vi "Basic TESTER.vi"() -> ()   [LabVIEW 2020]
uses:
  <vilib>/Rock Robotics/WPI/ThirdParty/Phoenix-LabVIEW/Pigeon IMU/CTRE_PigeonIMU_StatusFrameRate.ctl
  <vilib>/Rock Robotics/WPI/ThirdParty/Phoenix-LabVIEW/Pigeon IMU/CTRE_PigeonIMU_GetYPR.vi
  SwerveDrive/SwerveDrive_ACT.lvlib
  <vilib>/Rock Robotics/WPI/ThirdParty/Phoenix-LabVIEW/Pigeon2/controls/CTRE_Phoenix_Pigeon2_Configurables.ctl
  <vilib>/Rock Robotics/WPI/ThirdParty/Phoenix-LabVIEW/Pigeon IMU/CTRE_PigeonIMU_TareType.ctl
  Shared Code/TypeDefs/Dial_Compase heading unit circle CCW positive.ctl
panel:
  out "Yaw Angle":T1 scale format="%.3f"
  in  "Value":dbl format="%#_13g"
  in  "TareType (SetValue)":T2=2 items=["SetValue"=0, "AddOffset"=1, "MatchCompass"=2, "SetOffset"=255]
  in  "Set Yaw":bool
  out "error out":errorcluster
  out "periodMs":u32
  out "Has Reset Occurred?":bool
  out "Numeric":i32
  out "Yaw Pitch Roll":cluster{"Yaw":dbl, "Pitch":dbl, "Roll":dbl}
  out "firmware version":i32
  in  "Pigeon2 Configurables":T3
  in  "Finish":bool
  # "Pitch Angle needed to reach the current orientation in degrees"
  # "Yaw Angle needed to reach the current orientation in degrees"
  # "Configures the mounting pose of the Pigeon2\nThis is the yaw-pitch-roll teh Pigeon2 underwent to get to its current orientation,\n referenced from the robot's point of view\nThis is only necessary if the Pigeon2 is mounted at an exotic angle near the gimbal lock point or not forward.\nIf the pigeon is relatively flat and pointed forward, this is not needed"
  # "Roll Angle needed to reach the current orientation in degrees"
  # "Disables the temperature compensation\nfrom the Pigeon2. It is recommended that\nthis remains false"
  # "Disables the no-motion calibration from the\nPigeon2. It is recommended that this \nremains false"
  # "Enables the compass for Pigeon2\nThis is not recommended for any indoor robotics"
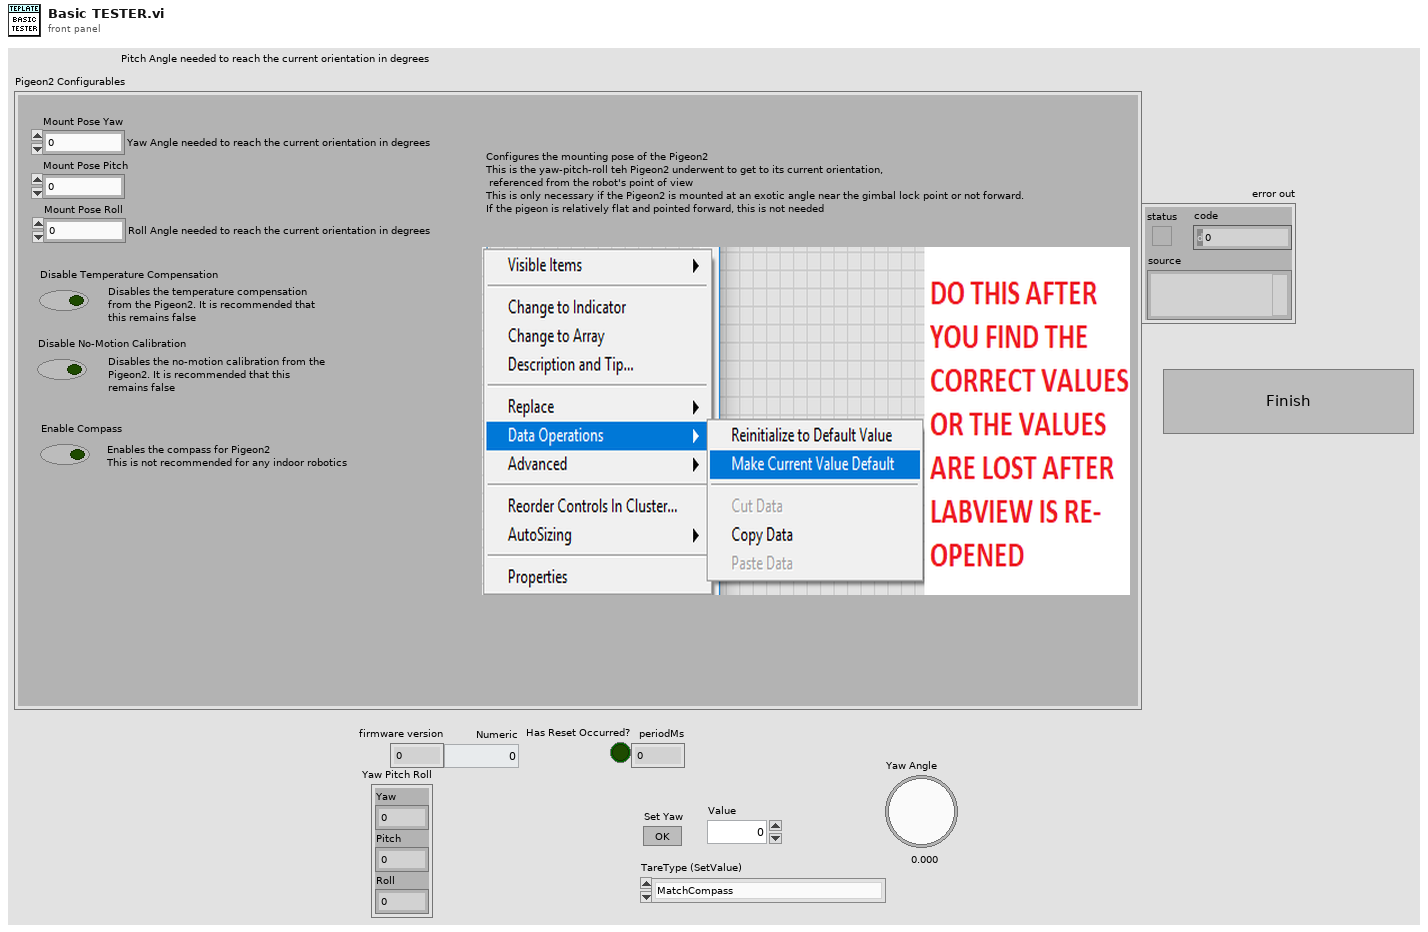
[diagram p1: front panel]
types:
  T1 = typedef "Dial_Compase heading unit circle CCW positive.ctl" = dbl
  T2 = typedef "CTRE_PigeonIMU_TareType.ctl" = u8
  T3 = typedef "CTRE_Phoenix_Pigeon2_Configurables.ctl" = cluster{"Mount Pose Yaw":dbl, "Mount Pose Pitch":dbl, "Mount Pose Roll":dbl, "Disable Temperature Compensation":bool, "Disable No-Motion Calibration":bool, "Enable Compass":bool}
  T4 = typedef "CTRE_PigeonIMU_DeviceRef.ctl" = cluster{"DeviceStatus":errorcluster, "Device Number":u8, "Type":T5, "Device ID":u32, "Handle":u64, "UsageFrame":u32, "Library Path":path}
  T5 = typedef "CTRE_PigeonIMU_ConnectionType.ctl" = u32
  T6 = typedef "CTRE_PigeonIMU_StatusFrameRate.ctl" = u32
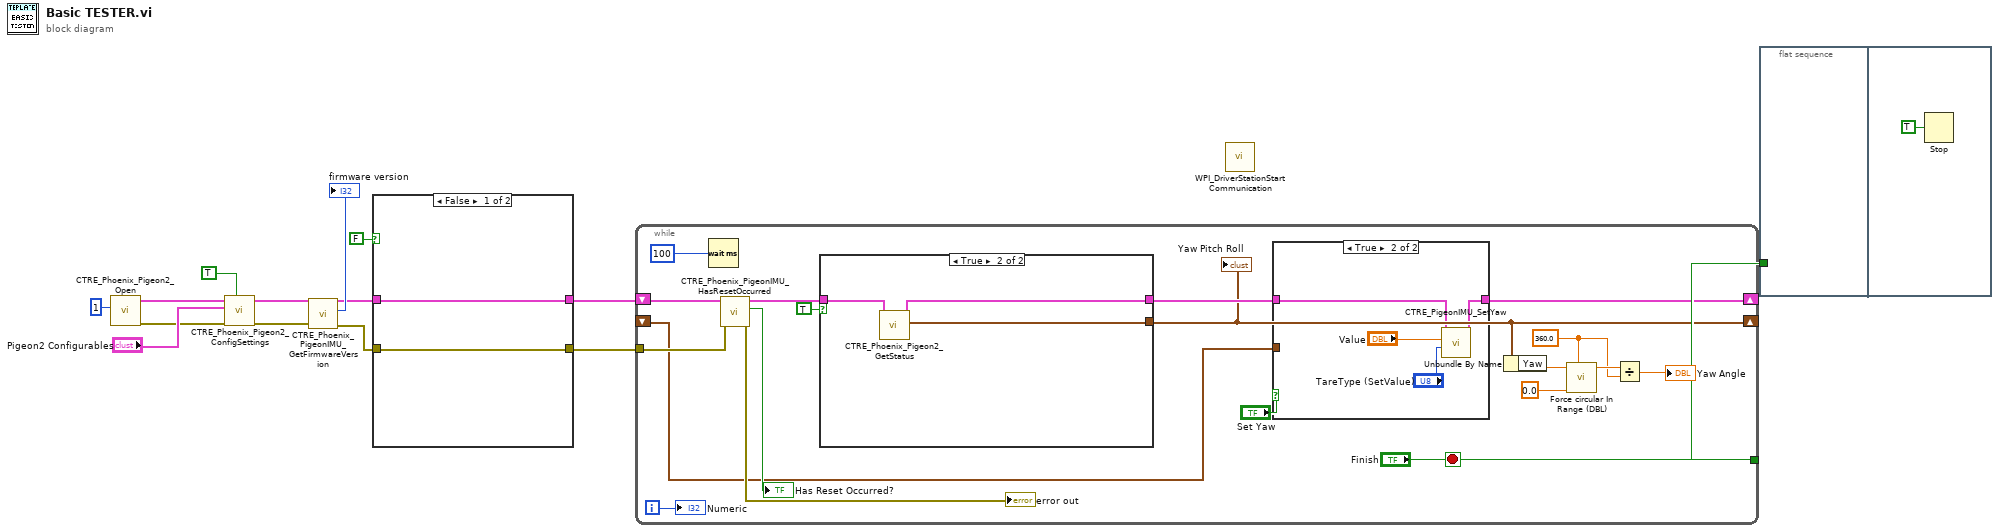
[diagram p0: block diagram]
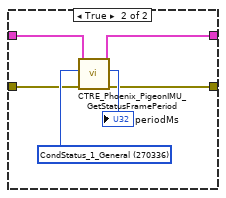
[diagram p2: hidden frame]
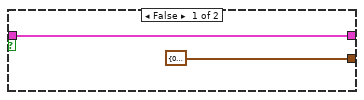
[diagram p4: hidden frame]
diagram:
  n1 = call <vilib>:"CTRE_Phoenix_Pigeon2_Open.vi"("Device Number"=u8 1) -> ("error out"=w5:errorcluster, "PigeonIMUDevRef"=w12:T4)  [unwired: 9 in]
  n2 = call <vilib>:"CTRE_Phoenix_Pigeon2_ConfigSettings.vi"("Force Write"=TRUE, "error in (no error)"=w5, "Pigeon2 Configurables"="Pigeon2 Configurables", "PigeonIMUDevRef 2"=w12) -> ("error out"=w4:errorcluster, "PigeonIMUDevRef"=w9:T4)  [unwired: 6 in]
  n3 = call <vilib>:"CTRE_Phoenix_PigeonIMU_GetFirmwareVersion.vi"("error in"=w4, "CTRE_PigeonIMU_DeviceRef"=w9) -> ("error out"=w3:errorcluster, "firmware version"=→"firmware version":i32, "CTRE_PigeonIMU_DeviceRef"=w7:T4)  [unwired: 7 in]
  n4 = case shown="False" FALSE {
    tunnel: w7 -> [w16 w22]
    tunnel: [w16 w21] -> w6
    tunnel: w3 -> [w15 w18]
    tunnel: [w15 w17] -> w2
    frame False {
    }
    frame True {
      w20 = T6 270336 items=["CondStatus_1_General"=270336, "CondStatus_9_SixDeg_YPR"=270848, "CondStatus_6_SensorFusion"=270656, "CondStatus_11_GyroAccum"=270976, "CondStatus_2_GeneralCompass"=270400, "CondStatus_3_GeneralAccel"=270464, "CondStatus_10_SixDeg_Quat"=270912, "RawStatus_4_Mag"=265408, "BiasedStatus_2_Gyro"=269376, "BiasedStatus_4_Mag"=269504, "BiasedStatus_6_Accel"=269632] ("Pigeon IMU Status Frame")
      n5 = call <vilib>:"CTRE_Phoenix_PigeonIMU_GetStatusFramePeriod.vi"("error in"=w18, "Pigeon IMU Status Frame"=w20, "CTRE_PigeonIMU_DeviceRef"=w22) -> ("error out"=w17:errorcluster, "periodMs"=→"periodMs":u32, "CTRE_PigeonIMU_DeviceRef"=w21:T4)  [unwired: 6 in]
    }
  }
  n6 = while {
    tunnel: ["Finish"] -> w14
    shift-right: [w31] -> _
    shift-left: w6 -> [w38]
    tunnel: w2 -> [w35]
    shift-right: [w28] -> _
    shift-left: _ -> [w29]
    i -> [w39]
    stop <- "Finish" stop-if-true
    w24 = 360.0 ("Max")
    n7 = Wait (ms)(milliseconds to wait=u32 100 ("Update Rate (ms)")) -> ()  [unwired: 1 out]
    n8 = call <vilib>:"CTRE_Phoenix_PigeonIMU_HasResetOccurred.vi"("error in"=w35, "CTRE_PigeonIMU_DeviceRef"=w38) -> ("error out"=→"error out":errorcluster, "Has Reset Occurred?"=→"Has Reset Occurred?":bool, "CTRE_PigeonIMU_DeviceRef"=w37:T4)  [unwired: 7 in]
    n9 = case shown="True" TRUE {
      tunnel: [w48 w51] -> w32
      tunnel: [cluster{"Yaw":dbl, "Pitch":dbl, "Roll":dbl} {"Yaw"=0.0, "Pitch"=0.0, "Roll"=0.0} ("Yaw Pitch Roll") w50] -> w28
      tunnel: w37 -> [w48 w49]
      frame False {
      }
      frame True {
        n10 = call-poly <vilib>:"CTRE_Phoenix_Pigeon2_GetStatus.vi"("PigeonIMUDevRef"=w49) -> ("Yaw Pitch Roll"=w50:cluster{"Yaw":dbl, "Pitch":dbl, "Roll":dbl}, "PigeonIMUDevRef"=w51:T4)  [unwired: 8 in, 1 out]
      }
    }
    "Yaw Pitch Roll" <- w28
    n11 = case shown="True" "Set Yaw" {
      tunnel: w32 -> [w42 w44]
      tunnel: [w42 w45] -> w31
      tunnel: w29 -> [_ _]
      frame False {
      }
      frame True {
        n12 = call <vilib>:"CTRE_PigeonIMU_SetYaw.vi"("TareType (SetValue)"="TareType (SetValue)", "Value"="Value", "PigeonIMUDevRef"=w44) -> ("PigeonIMUDevRef"=w45:T4)  [unwired: 7 in, 1 out]
      }
    }
    n13 = Unbundle By Name(w28) -> ("Yaw"=w27:dbl)
    n14 = call "Force circular In Range (DBL).vi"("Max"=w24, "Min"=0.0, "Value"=w27) -> ("Value Out"=w25:dbl)  [unwired: 7 in, 1 out]
    n15 = Divide(x=w25, y=w24) -> (x/y=→"Yaw Angle":dbl)
    "Numeric" <- w39
  }
  n16 = call <vilib>:"WPI_DriverStationStart Communication.vi"() -> ()  [unwired: 3 in, 9 out]
  n17 = flat-sequence {
    tunnel: w14 -> [_]
    frame #0 {
    }
    frame #1 {
      n18 = Stop(stop? (T)=TRUE) -> ()
    }
  }
